vi "GoToGuardPosition.vi"(8 "error in (no error)":errorcluster, 11 "object in":refnum<class "GoToSkill_v2.lvclass">) -> (0 "error out":errorcluster, 3 "object out":refnum<class "GoToSkill_v2.lvclass">)   [LabVIEW 2023, in "GoToSkill_v2.lvclass"]
uses:
  GoToSkill_v2.lvclass
  Robot_class/Robot.lvclass
  Ball_class/Ball.lvclass
  C:/Users/ebert/Documents/codes/SSL/repo/SSL_AI/Object_class/Object.lvclass
  Object_class/Object.lvclass/Object.ctl
  Object_class/Read position(x,y).vi
  Zone_class/Zone.lvclass
panel:
  out "Robot out":refnum<class "Robot.lvclass">
  in  "Ball":refnum<class "Ball.lvclass">
  in  "Robot":refnum<class "Robot.lvclass">
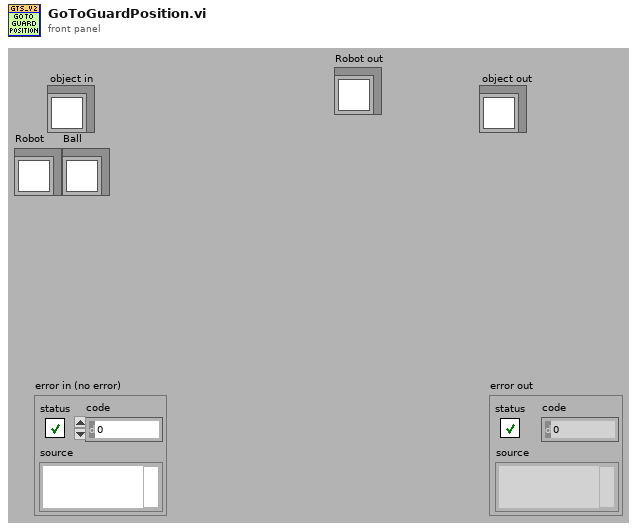
[diagram p1: front panel]
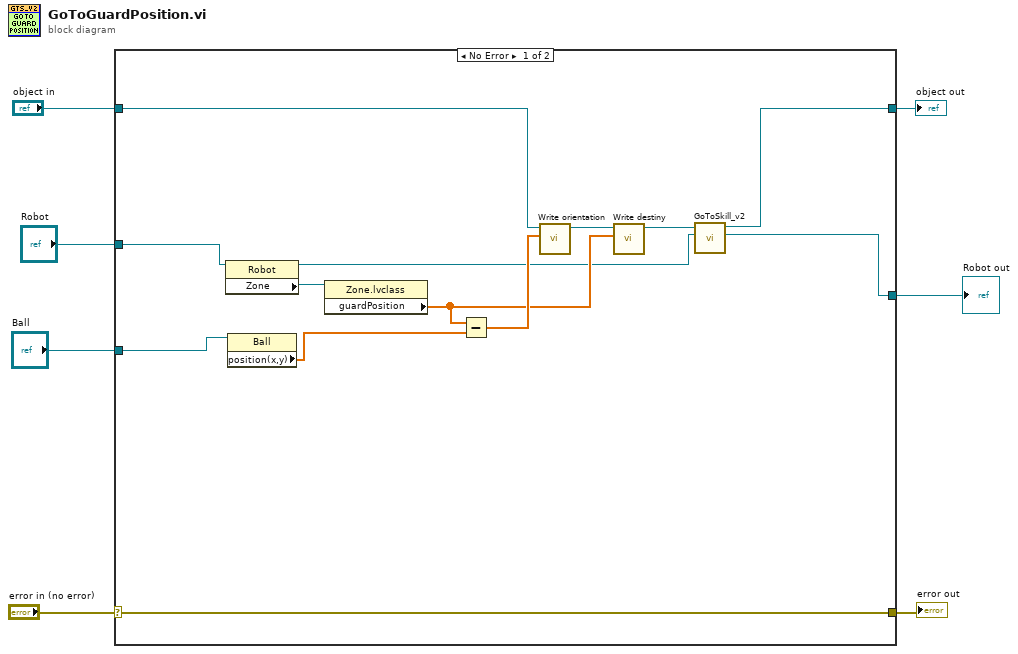
[diagram p0: block diagram]
diagram:
  n1 = case shown="No Error" "error in (no error)" {
    selector: "error in (no error)" -> [w20 w23]
    tunnel: [w20 w23] -> w6
    tunnel: [w9 w22] -> w4
    tunnel: "object in" -> [w10 w22]
    tunnel: "Ball" -> [w12 _]
    tunnel: "Robot" -> [w11 w21]
    tunnel: [w8 w21] -> w1
    frame No Error {
      n2 = property class="Robot"(reference=w11) -> (reference out=w13:refnum<class "Robot.lvclass">, "Zone"=w17:refnum<class "Zone.lvclass">)  [unwired: 1 in, 1 out]
      n3 = property class="Ball"(reference=w12) -> ("position(x,y)"=w16:dbl[])  [unwired: 1 in, 2 out]
      n4 = property class="Zone.lvclass"(reference=w17) -> ("guardPosition"=w14:dbl[])  [unwired: 1 in, 2 out]
      n5 = Subtract(x=w14, y=w16) -> (x-y=w15:dbl[])
      n6 = call-dynamic "Write orientation.vi"("orientation"=w15, "GoToSkill_v2 in"=w10) -> ("GoToSkill_v2 out"=w19:refnum<class "GoToSkill_v2.lvclass">)  [unwired: 8 in, 1 out]
      n7 = call-dynamic "Write destiny.vi"("destiny"=w14, "GoToSkill_v2 in"=w19) -> ("GoToSkill_v2 out"=w18:refnum<class "GoToSkill_v2.lvclass">)  [unwired: 8 in, 1 out]
      n8 = call-dynamic "GoToSkill_v2.vi"("Robot"=w13, "object in"=w18) -> ("Robot out"=w8:refnum<class "Robot.lvclass">, "object out"=w9:refnum<class "GoToSkill_v2.lvclass">)  [unwired: 7 in, 1 out]
    }
    frame Error {
    }
  }
  "error out" <- w6
  "object out" <- w4
  "Robot out" <- w1
